vi "Publish ViewModel Data.vi"(8 "error in (no error)":errorcluster, 9 "Data to Publish":variant, 10 "Datum Name":string, 11 "IViewModel In":refnum<class "IViewModel.lvclass">) -> (0 "error out":errorcluster, 3 "IViewModel Out":refnum<class "IViewModel.lvclass">)   [LabVIEW 2015, in "IViewModel.lvlib" / "IViewModel.lvclass"]
doc: "<License>\nCopyright © 2017 Composed Systems, LLC | All rights reserved\nwww.composed.io\n\nAuthor: Ethan Stern <ethan.stern@composed.io>\n\nThis software is provided \"AS IS\" WITHOUT WARRANTIES, either express or implied, AND IS FOR EDUCATIONAL PURPOSES ONLY.\n</License>"
uses:
  IViewModel.lvclass
  IViewModel.lvclass/IViewModel.ctl
  IMediator/IMediator Messages/Publish Msg/Publish Msg.lvclass/Publish Msg.ctl
  <vilib>/ActorFramework/Message Enqueuer/Message Enqueuer.lvclass/Message Enqueuer.ctl
  <vilib>/ActorFramework/Message Enqueuer/Enqueue.vi
  <vilib>/ActorFramework/Message Priority Queue/Priority Enqueue.vi
  IMediator/IMediator Messages/Publish Msg/Publish Msg.lvclass
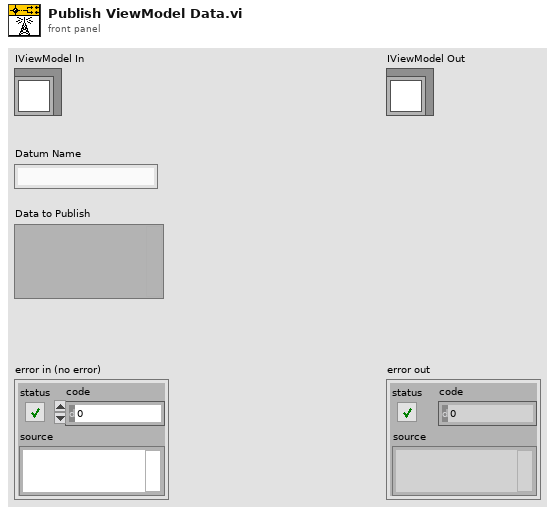
[diagram p1: front panel]
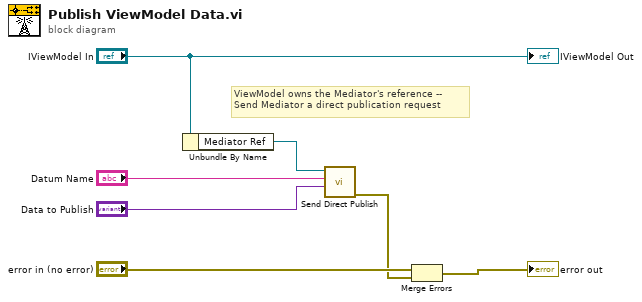
[diagram p0: block diagram]
diagram:
  # "ViewModel owns the Mediator's reference --\nSend Mediator a direct publication request"
  n1 = Unbundle By Name("IViewModel In") -> ("Mediator Ref"=w6:refnum<class "Message Enqueuer.lvclass">)
  n2 = call "Send Direct Publish.vi"("Data to Publish"="Data to Publish", "Topic Name"="Datum Name", "Mediator Enqeuer"=w6) -> ("error out"=w1:errorcluster)  [unwired: 7 in, 1 out]
  n3 = Merge Errors("error in (no error)", w1) -> (→"error out":errorcluster)
  "IViewModel Out" <- "IViewModel In"
